vi "FS50_auto-tune_LV2019.vi"() -> ()   [LabVIEW 2019]
uses:
  C/Program Files (x86)/National Instruments/LabVIEW 2021/instr.lib/NKTP_API/NKTP_API.lvlib
panel:
  out "Auto-tune Status":string
  out "Current D4":dbl
  out "Current D3":dbl
  out "Current D2":dbl
  out "Connected":bool
  in  "Auto-tune":bool
  out "Auto-tune on":bool
  in  "Power Level":u16(slide) max=100 step=1 scale=0.0..100.0
  out "Emission On":bool
  in  "Emission":bool
  in  "VISA resource name":refnum<visa-resource-name>
  in  "Exit":bool
  in  "Connect":bool
  out "error out":errorcluster
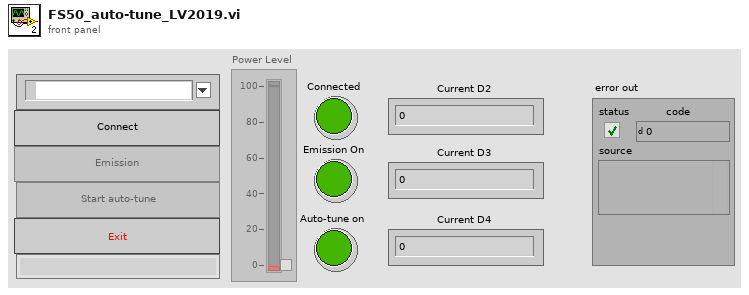
[diagram p1: front panel]
types:
  T1 = enum8{"Enabled", "Disabled", "Disabled and Grayed Out"}
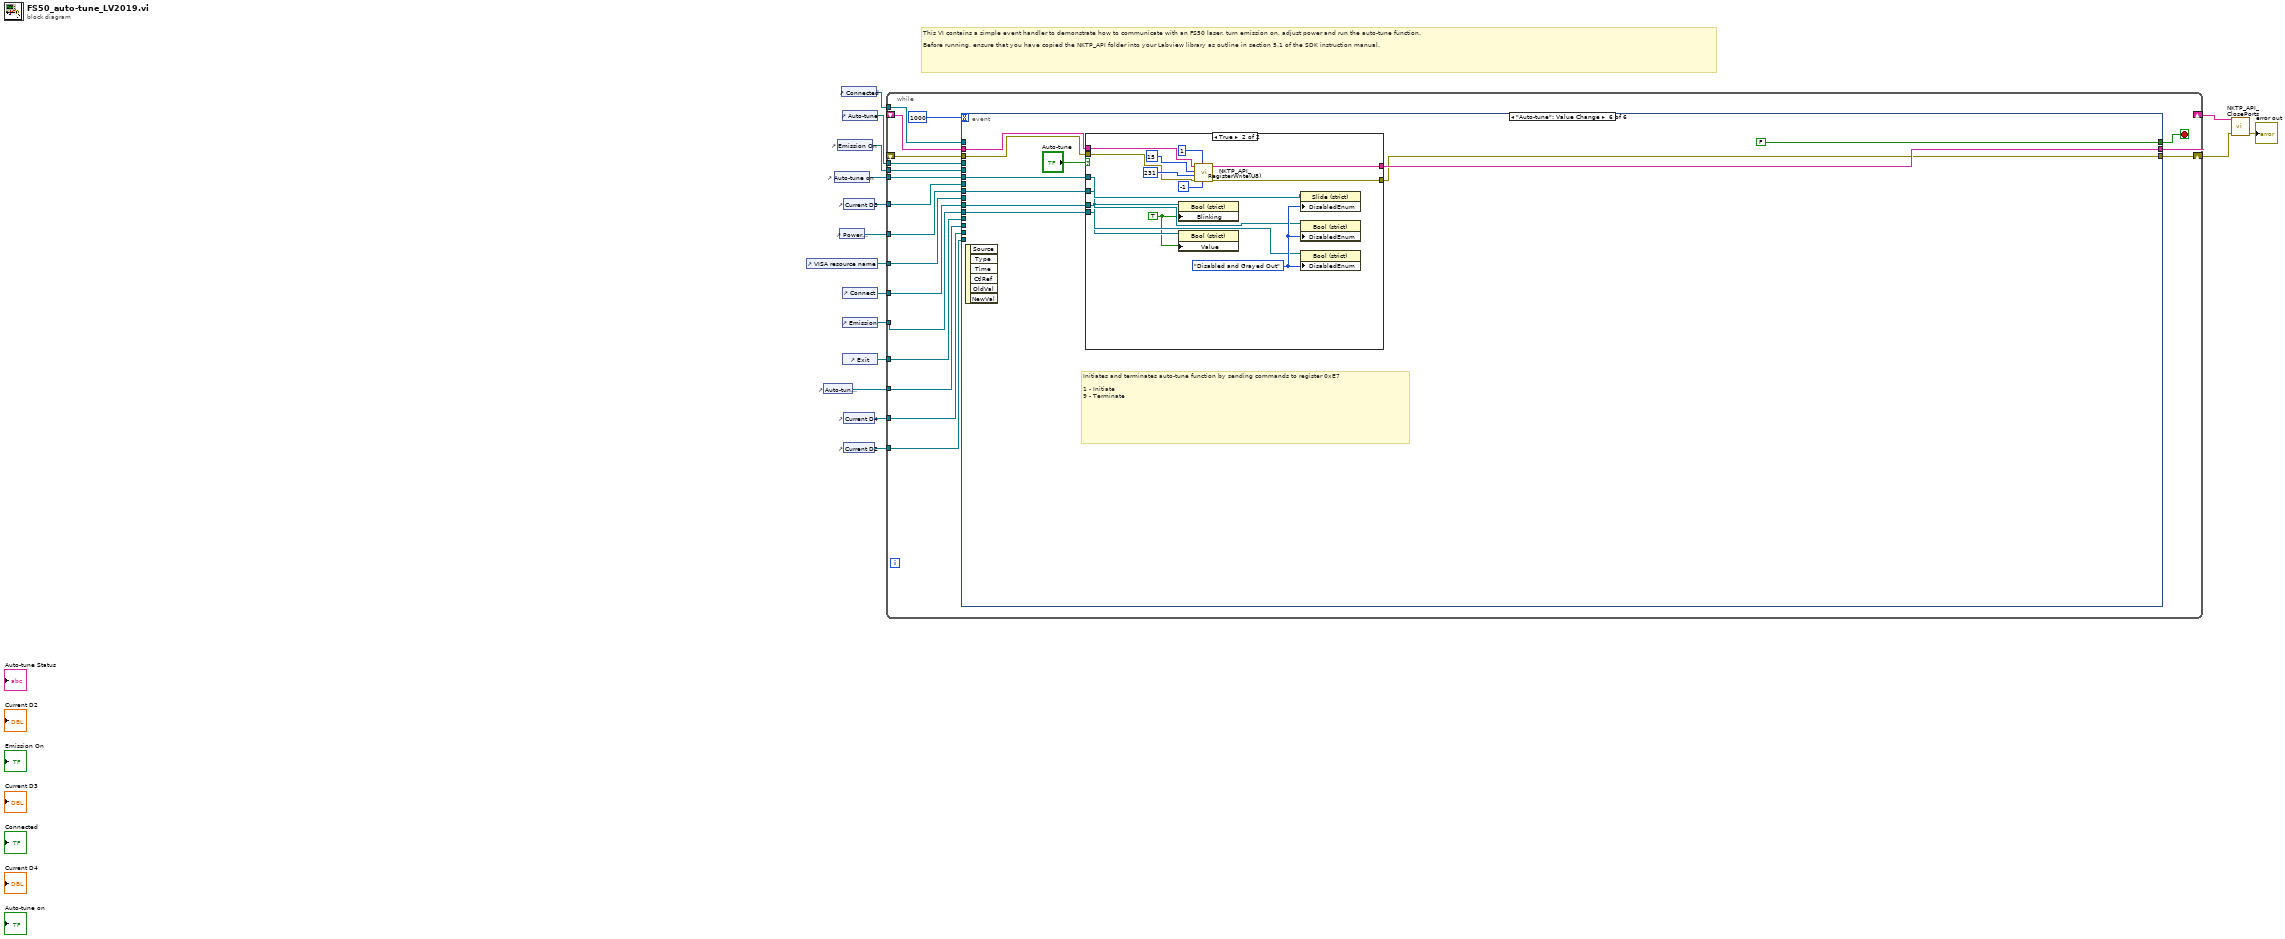
[diagram p0: block diagram]
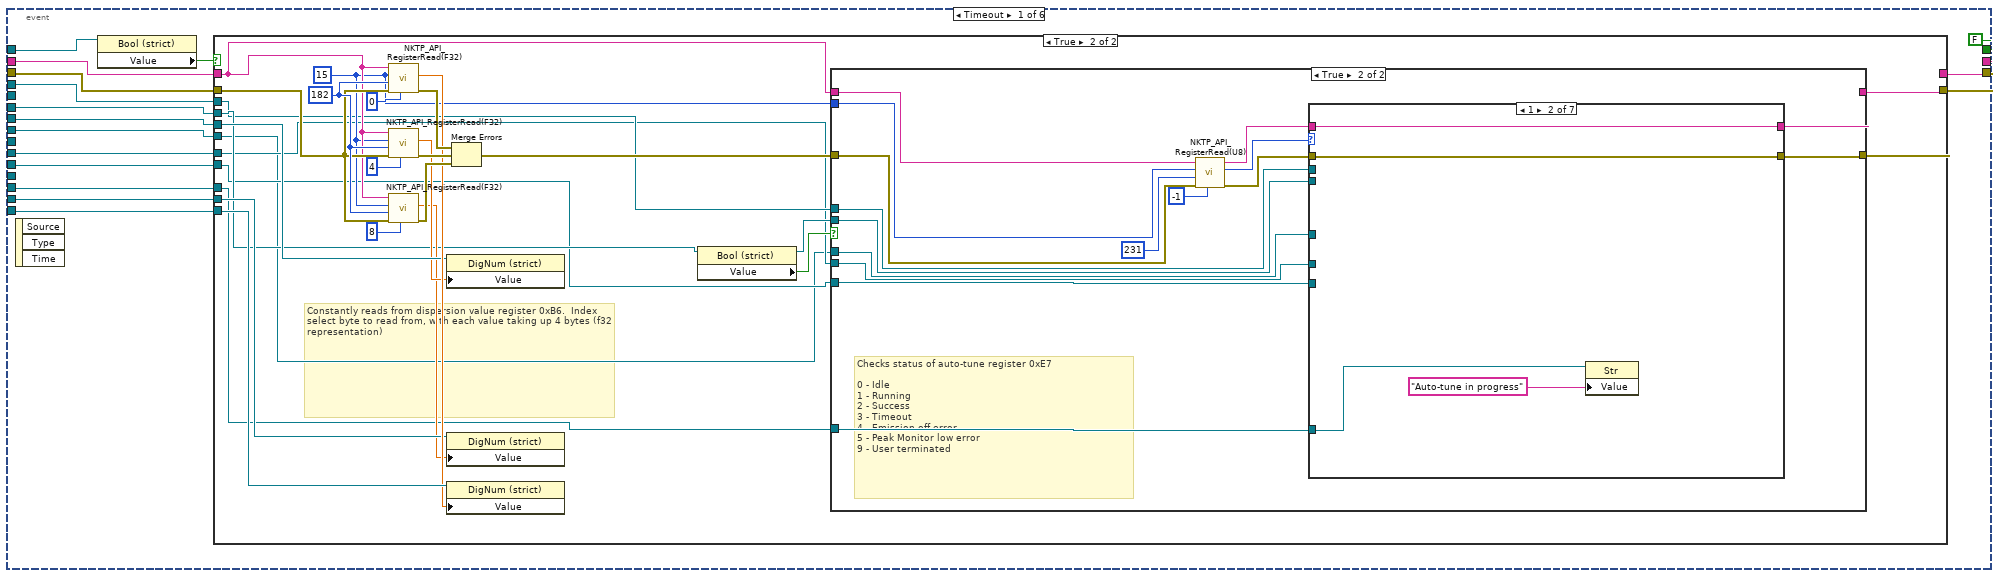
[diagram p2: hidden frame]
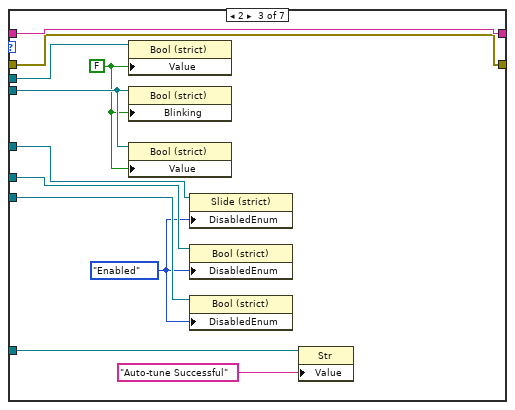
[diagram p6: hidden frame]
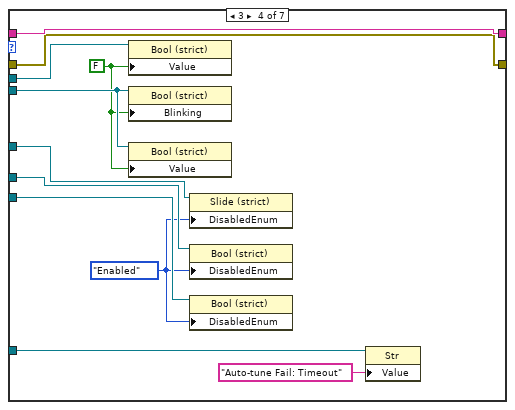
[diagram p7: hidden frame]
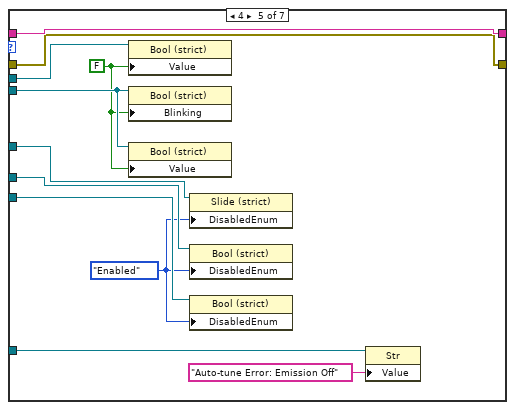
[diagram p8: hidden frame]
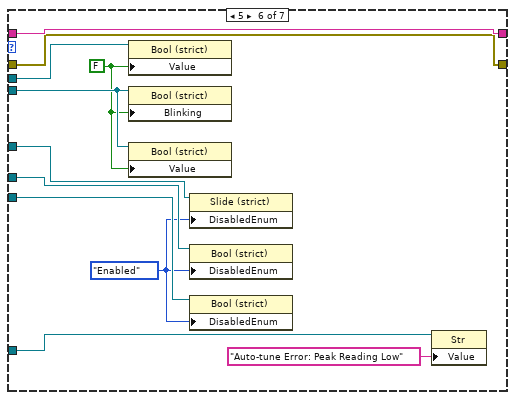
[diagram p9: hidden frame]
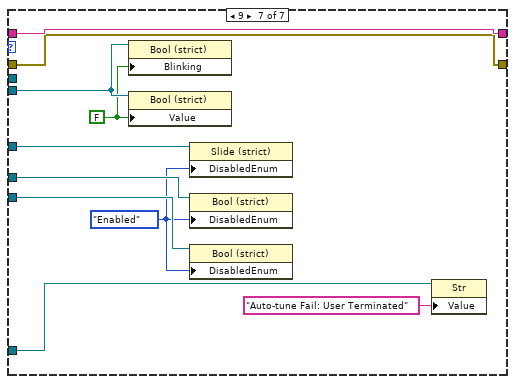
[diagram p10: hidden frame]
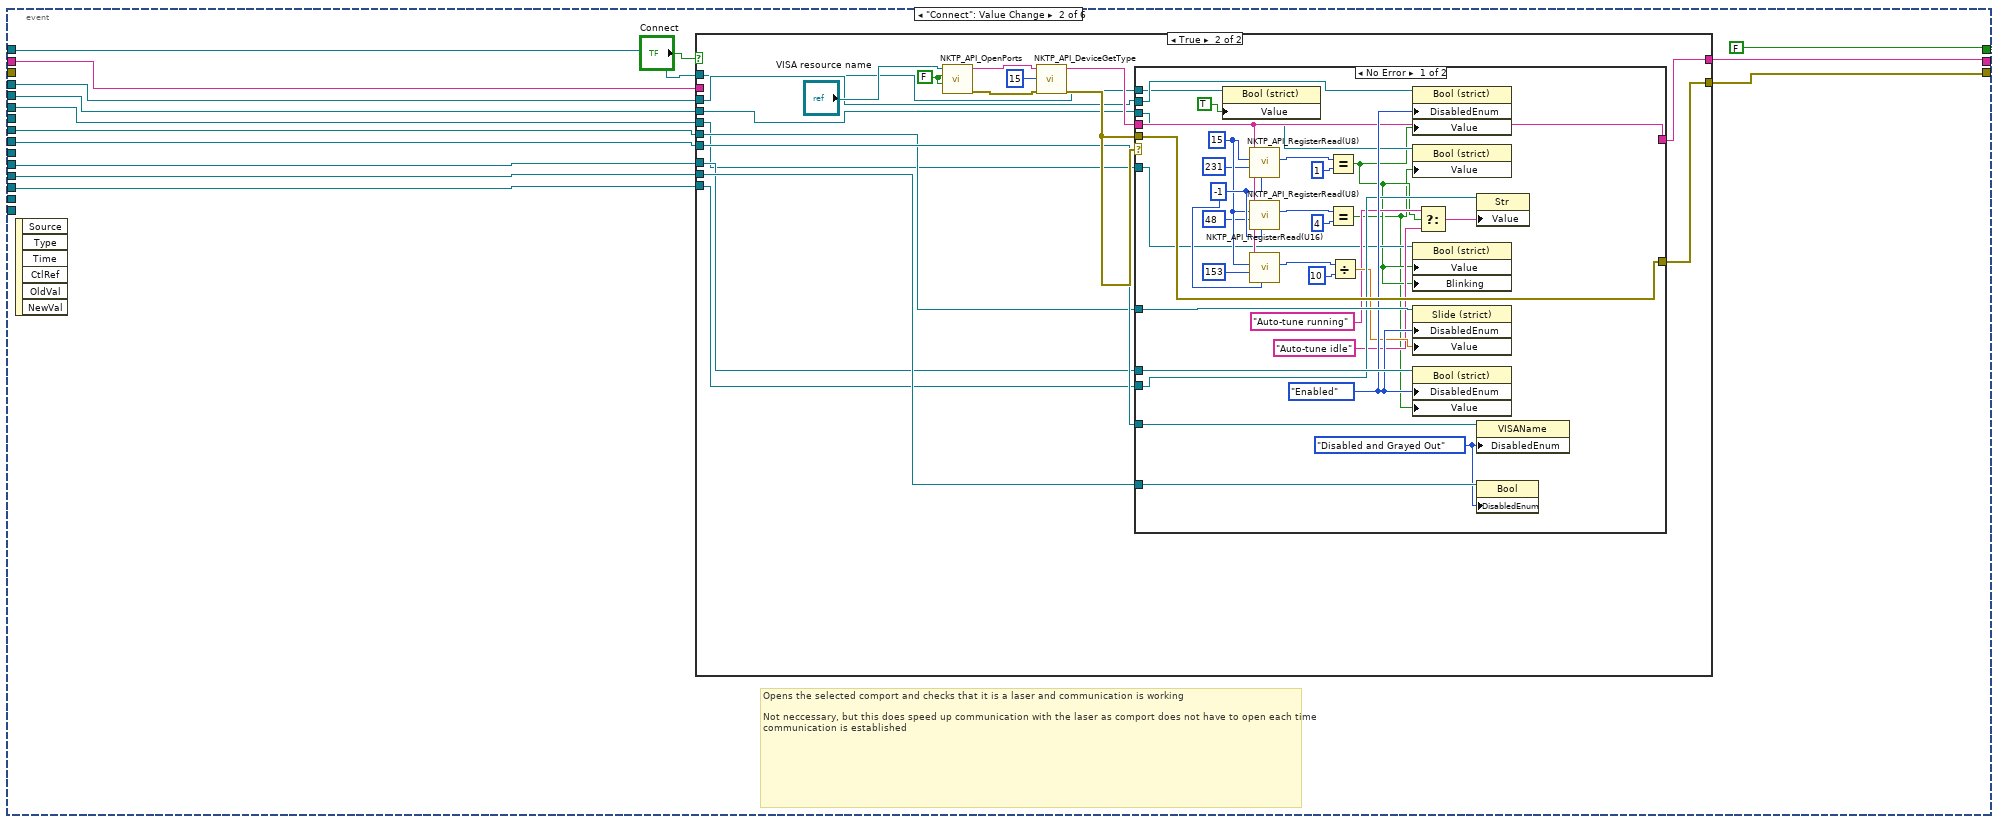
[diagram p11: hidden frame]
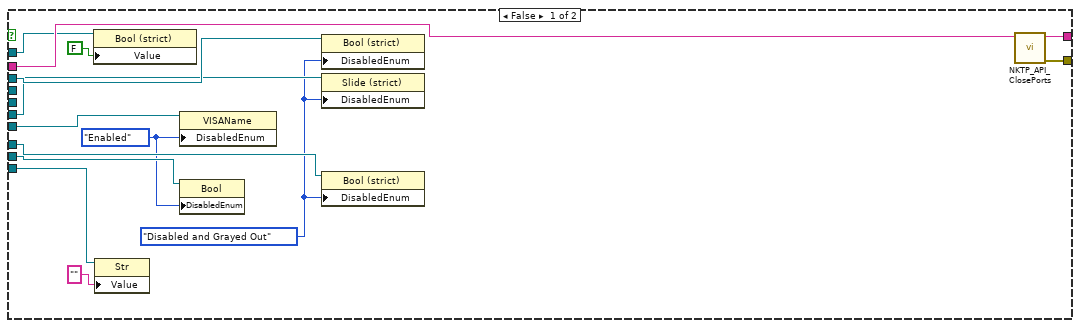
[diagram p12: hidden frame]
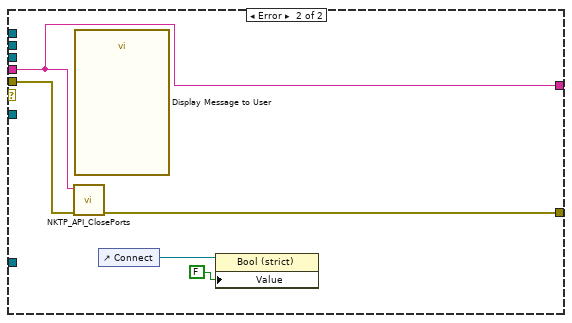
[diagram p13: hidden frame]
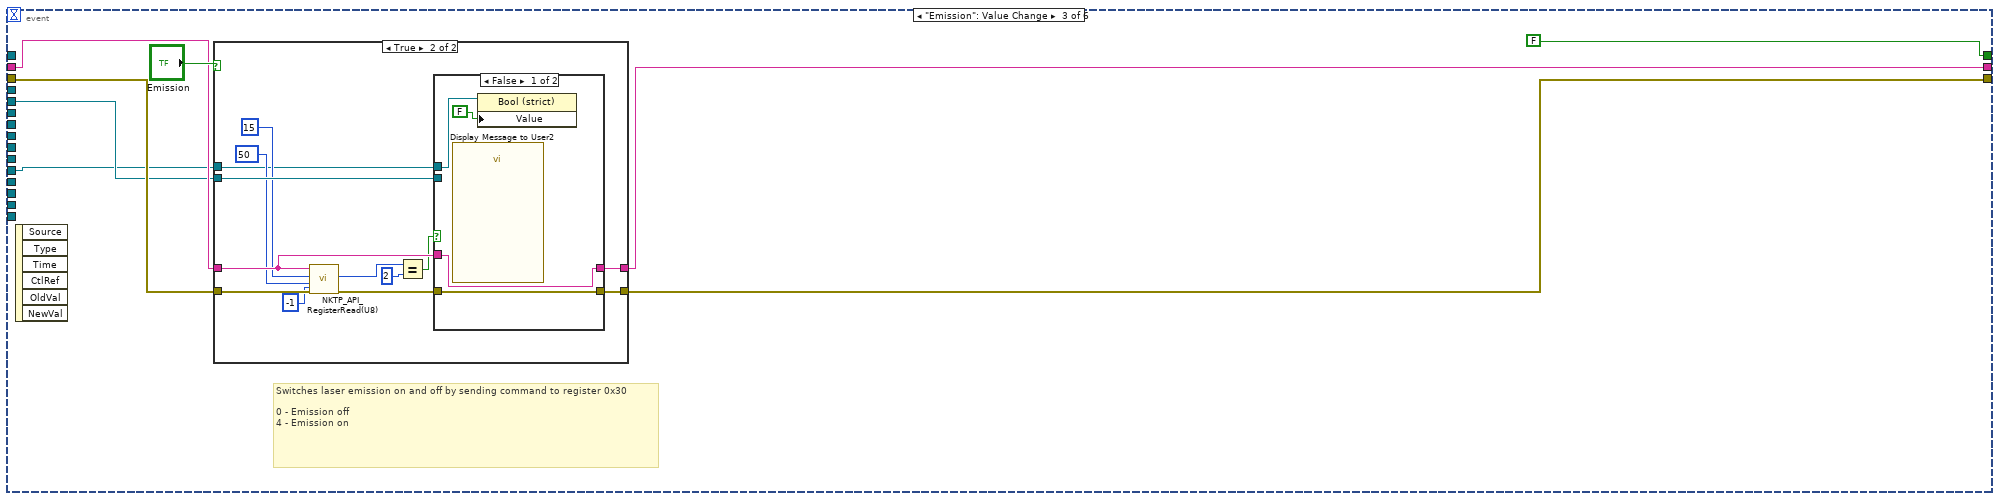
[diagram p14: hidden frame]
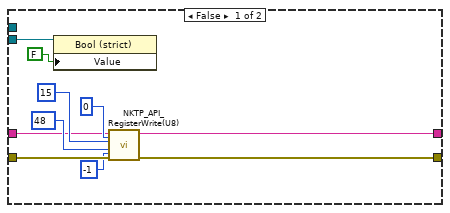
[diagram p15: hidden frame]
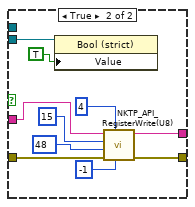
[diagram p16: hidden frame]
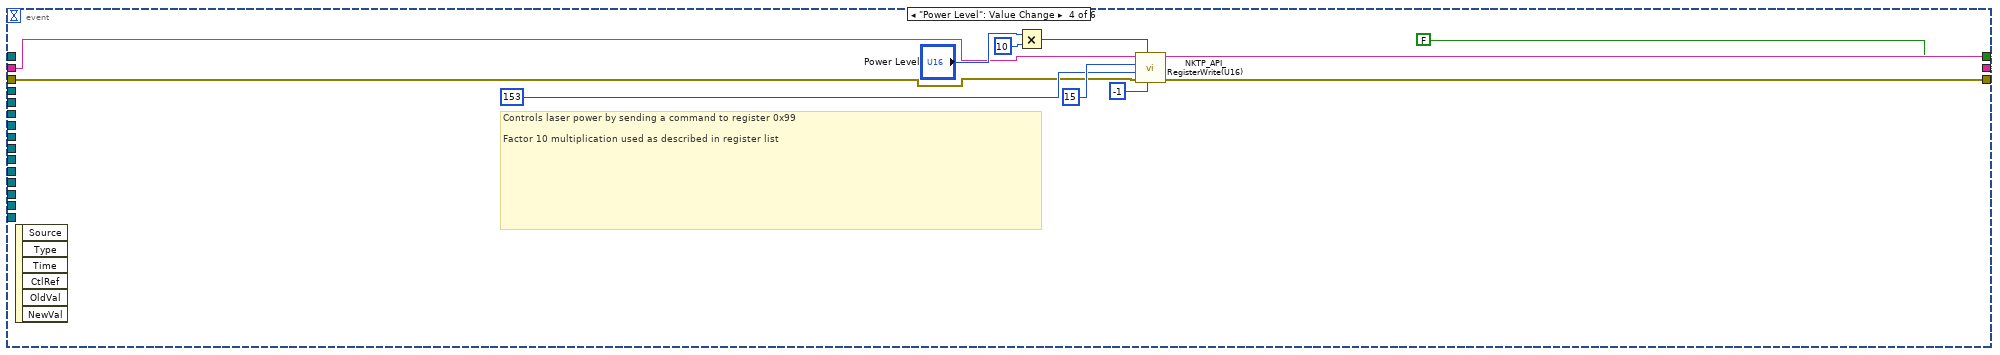
[diagram p17: hidden frame]
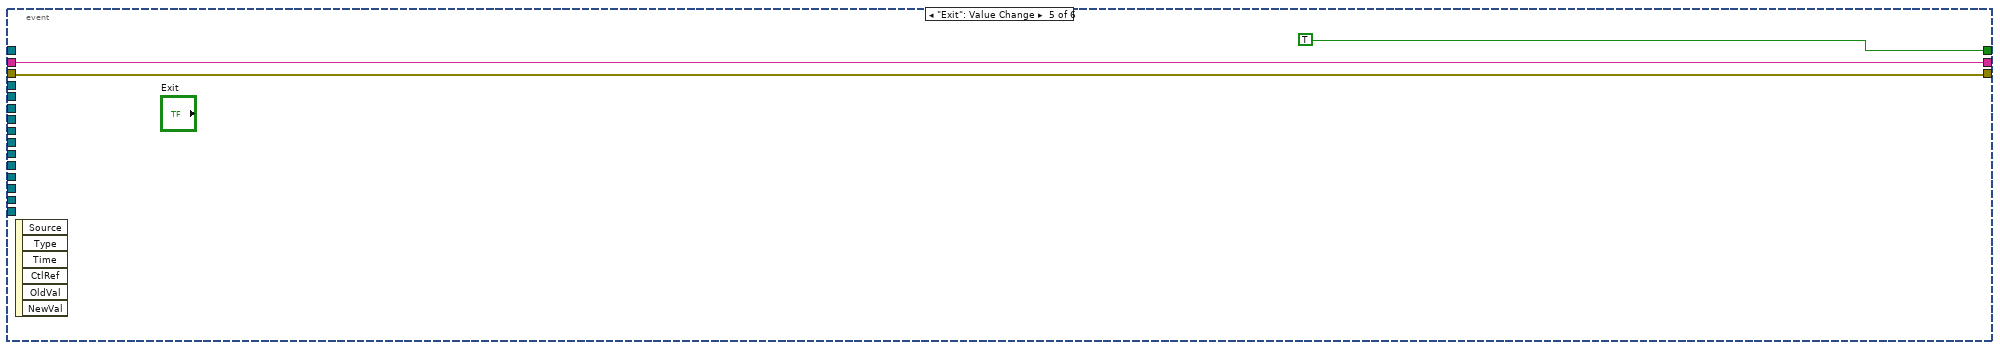
[diagram p18: hidden frame]
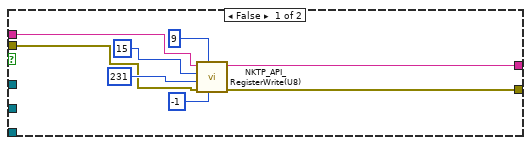
[diagram p19: hidden frame]
diagram:
  # "This VI contains a simple event handler to demonstrate how to communicate with an FS50 laser, turn emission on, adjust power and run the auto-tune function.\n\nBefore running, ensure that you have copied the NKTP_API folder into your Labview library as outline in section 5.1 of the SDK instruction manual."
  n1 = control-ref of="VISA resource name"() -> (w9:refnum<vi>)
  n2 = control-ref of="Auto-tune Status"() -> (w1:refnum<vi>)
  n3 = control-ref of="Auto-tune on"() -> (w13:refnum<vi>)
  n4 = control-ref of="Emission On"() -> (w7:refnum<vi>)
  n5 = control-ref of="Power Level"() -> (w10:refnum<vi>)
  n6 = control-ref of="Connected"() -> (w6:refnum<vi>)
  n7 = control-ref of="Auto-tune"() -> (w12:refnum<vi>)
  n8 = control-ref of="Connect"() -> (w2:refnum<vi>)
  n9 = control-ref of="Emission"() -> (w11:refnum<vi>)
  n10 = control-ref of="Exit"() -> (w8:refnum<vi>)
  n11 = control-ref of="Current D3"() -> (w4:refnum<vi>)
  n12 = control-ref of="Current D4"() -> (w3:refnum<vi>)
  n13 = control-ref of="Current D2"() -> (w5:refnum<vi>)
  n14 = while {
    shift-right: [w33] -> w14
    shift-left: _ -> [w30]
    shift-right: [w35] -> w16
    shift-left: _ -> [w32]
    tunnel: w13 -> [w29]
    tunnel: w12 -> [w28]
    tunnel: w11 -> [w27]
    tunnel: w10 -> [w26]
    tunnel: w9 -> [w25]
    tunnel: w8 -> [w24]
    tunnel: w7 -> [w23]
    tunnel: w6 -> [w22]
    tunnel: w5 -> [w21]
    tunnel: w4 -> [w20]
    tunnel: w3 -> [w19]
    tunnel: w2 -> [w18]
    tunnel: w1 -> [w17]
    stop <- w34 stop-if-true
    n15 = event shown="[5] \"Auto-tune\": Value Change" {
      selector: _ -> [_ _ _ _ _ _]
      dyn-events: _ -> [_ _ _ _ _ _]
      timeout: 1000 -> [_ _ _ _ _ _]
      tunnel: [w48 w172 w245 w289 w297 w301] -> w33
      tunnel: [w47 w171 w244 w290 w298 w303] -> w35
      tunnel: [FALSE FALSE FALSE FALSE TRUE FALSE] -> w34
      tunnel: w32 -> [w46 w168 w247 w293 w298 w307]
      tunnel: w30 -> [w51 _ w246 w288 w297 w302]
      tunnel: w29 -> [w42 w159 _ _ _ w308]
      tunnel: w28 -> [w40 w167 _ _ _ _]
      tunnel: w27 -> [w38 w166 w241 _ _ w306]
      tunnel: w26 -> [w37 w165 _ _ _ w304]
      tunnel: w25 -> [_ w164 _ _ _ _]
      tunnel: w24 -> [_ w163 _ _ _ _]
      tunnel: w23 -> [_ w160 w243 _ _ _]
      tunnel: w22 -> [w50 w162 _ _ _ _]
      tunnel: w21 -> [w45 _ _ _ _ _]
      tunnel: w20 -> [w44 _ _ _ _ _]
      tunnel: w19 -> [w43 _ _ _ _ _]
      tunnel: w18 -> [w39 _ _ _ _ w305]
      tunnel: w17 -> [w41 w161 _ _ _ _]
      event Timeout {
        n16 = event-data() -> ()  [unwired: 1 in, 3 out]
        n17 = property class="Bool (strict)"(reference=w50) -> ("Value"=w49:bool)  [unwired: 1 in, 2 out]
        n18 = case shown="True" w49 {
          tunnel: w51 -> [w53 w79]
          tunnel: [w53 w61] -> w48
          tunnel: [w52 w60] -> w47
          tunnel: w46 -> [w52 w64]
          tunnel: w45 -> [_ w72]
          tunnel: w44 -> [_ w70]
          tunnel: w43 -> [_ w68]
          tunnel: w42 -> [_ w66]
          tunnel: w41 -> [_ w59]
          tunnel: w40 -> [_ w57]
          tunnel: w39 -> [_ w56]
          tunnel: w38 -> [_ w55]
          tunnel: w37 -> [_ w54]
          frame False {
          }
          frame True {
            w80 = u8 182 ("regId")
            w63 = u8 15 ("devId")
            # "Constantly reads from dispersion value register 0xB6.  Index select byte to read from, with each value taking up 4 bytes (f32 representation)"
            n19 = call <instrlib>:"NKTP_API_RegisterRead(F32).vi"("index"=i16 0, "error in"=w79, "regId"=w80, "devId"=w63, "portname"=w64) -> ("error out"=w78:errorcluster, "value"=w71:sgl)  [unwired: 4 in, 1 out]
            n20 = call <instrlib>:"NKTP_API_RegisterRead(F32).vi"("index"=i16 4, "error in"=w79, "regId"=w80, "devId"=w63, "portname"=w64) -> ("error out"=w77:errorcluster, "value"=w69:sgl)  [unwired: 4 in, 1 out]
            n21 = call <instrlib>:"NKTP_API_RegisterRead(F32).vi"("index"=i16 8, "error in"=w79, "regId"=w80, "devId"=w63, "portname"=w64) -> ("error out"=w76:errorcluster, "value"=w67:sgl)  [unwired: 4 in, 1 out]
            n22 = property class="DigNum (strict)"(reference=w70, "Value"=w69) -> ()  [unwired: 1 in, 2 out]
            n23 = property class="DigNum (strict)"(reference=w68, "Value"=w67) -> ()  [unwired: 1 in, 2 out]
            n24 = property class="DigNum (strict)"(reference=w72, "Value"=w71) -> ()  [unwired: 1 in, 2 out]
            n25 = Merge Errors(w78, w77, w76) -> (w62:errorcluster)
            n26 = property class="Bool (strict)"(reference=w66) -> (reference out=w58:refnum<vi>, "Value"=w65:bool)  [unwired: 1 in, 1 out]
            n27 = case shown="True" w65 {
              tunnel: w64 -> [w81 w98]
              tunnel: w63 -> [_ w97]
              tunnel: w62 -> [w82 w94]
              tunnel: [w82 w88] -> w61
              tunnel: [w81 w90] -> w60
              tunnel: w59 -> [_ w92]
              tunnel: w58 -> [_ w87]
              tunnel: w57 -> [_ w86]
              tunnel: w56 -> [_ w85]
              tunnel: w55 -> [_ w84]
              tunnel: w54 -> [_ w83]
              frame False {
              }
              frame True {
                # "Checks status of auto-tune register 0xE7\n\n0 - Idle\n1 - Running\n2 - Success\n3 - Timeout\n4 - Emission off error\n5 - Peak Monitor low error\n9 - User terminated"
                n28 = call <instrlib>:"NKTP_API_RegisterRead(U8).vi"("index"=i16 -1, "error in"=w94, "regId"=u8 231, "devId"=w97, "portname"=w98) -> ("error out"=w89:errorcluster, "value"=w93:u8, "portname out"=w91:string)  [unwired: 4 in]
                n29 = case shown="1" w93 {
                  tunnel: w92 -> [_ w104 w115 w126 w137 w148 w158]
                  tunnel: w91 -> [w100 w102 w113 w124 w135 w146 w156]
                  tunnel: [w100 w102 w113 w124 w135 w146 w156] -> w90
                  tunnel: w89 -> [w99 w101 w112 w123 w134 w145 w155]
                  tunnel: [w99 w101 w112 w123 w134 w145 w155] -> w88
                  tunnel: w87 -> [_ _ w106 w117 w128 w139 w150]
                  tunnel: w86 -> [_ _ w111 w122 w133 w144 _]
                  tunnel: w85 -> [_ _ w110 w121 w132 w143 w154]
                  tunnel: w84 -> [_ _ w109 w120 w131 w142 w153]
                  tunnel: w83 -> [_ _ w108 w119 w130 w141 w152]
                  frame 0, Default {
                  }
                  frame 1 {
                    n30 = property class="Str"(reference=w104, "Value"="Auto-tune in progress") -> ()  [unwired: 1 in, 2 out]
                  }
                  frame 2 {
                    w107 = T1."Enabled" ("Disabled")
                    w105 = FALSE ("Value")
                    n31 = property class="Bool (strict)"(reference=w111, "Value"=w105) -> ()  [unwired: 1 in, 2 out]
                    n32 = property class="Bool (strict)"(reference=w106, "Blinking"=w105) -> ()  [unwired: 1 in, 2 out]
                    n33 = property class="Bool (strict)"(reference=w106, "Value"=w105) -> ()  [unwired: 1 in, 2 out]
                    n34 = property class="Slide (strict)"(reference=w108, "DisabledEnum"=w107) -> ()  [unwired: 1 in, 2 out]
                    n35 = property class="Bool (strict)"(reference=w110, "DisabledEnum"=w107) -> ()  [unwired: 1 in, 2 out]
                    n36 = property class="Bool (strict)"(reference=w109, "DisabledEnum"=w107) -> ()  [unwired: 1 in, 2 out]
                    n37 = property class="Str"(reference=w115, "Value"="Auto-tune Successful") -> ()  [unwired: 1 in, 2 out]
                  }
                  frame 3 {
                    w118 = T1."Enabled" ("Disabled")
                    w116 = FALSE ("Value")
                    n38 = property class="Bool (strict)"(reference=w122, "Value"=w116) -> ()  [unwired: 1 in, 2 out]
                    n39 = property class="Bool (strict)"(reference=w117, "Blinking"=w116) -> ()  [unwired: 1 in, 2 out]
                    n40 = property class="Bool (strict)"(reference=w117, "Value"=w116) -> ()  [unwired: 1 in, 2 out]
                    n41 = property class="Slide (strict)"(reference=w119, "DisabledEnum"=w118) -> ()  [unwired: 1 in, 2 out]
                    n42 = property class="Bool (strict)"(reference=w121, "DisabledEnum"=w118) -> ()  [unwired: 1 in, 2 out]
                    n43 = property class="Bool (strict)"(reference=w120, "DisabledEnum"=w118) -> ()  [unwired: 1 in, 2 out]
                    n44 = property class="Str"(reference=w126, "Value"="Auto-tune Fail: Timeout") -> ()  [unwired: 1 in, 2 out]
                  }
                  frame 4 {
                    w129 = T1."Enabled" ("Disabled")
                    w127 = FALSE ("Value")
                    n45 = property class="Bool (strict)"(reference=w133, "Value"=w127) -> ()  [unwired: 1 in, 2 out]
                    n46 = property class="Bool (strict)"(reference=w128, "Blinking"=w127) -> ()  [unwired: 1 in, 2 out]
                    n47 = property class="Bool (strict)"(reference=w128, "Value"=w127) -> ()  [unwired: 1 in, 2 out]
                    n48 = property class="Slide (strict)"(reference=w130, "DisabledEnum"=w129) -> ()  [unwired: 1 in, 2 out]
                    n49 = property class="Bool (strict)"(reference=w132, "DisabledEnum"=w129) -> ()  [unwired: 1 in, 2 out]
                    n50 = property class="Bool (strict)"(reference=w131, "DisabledEnum"=w129) -> ()  [unwired: 1 in, 2 out]
                    n51 = property class="Str"(reference=w137, "Value"="Auto-tune Error: Emission Off") -> ()  [unwired: 1 in, 2 out]
                  }
                  frame 5 {
                    w140 = T1."Enabled" ("Disabled")
                    w138 = FALSE ("Value")
                    n52 = property class="Bool (strict)"(reference=w144, "Value"=w138) -> ()  [unwired: 1 in, 2 out]
                    n53 = property class="Bool (strict)"(reference=w139, "Blinking"=w138) -> ()  [unwired: 1 in, 2 out]
                    n54 = property class="Bool (strict)"(reference=w139, "Value"=w138) -> ()  [unwired: 1 in, 2 out]
                    n55 = property class="Slide (strict)"(reference=w141, "DisabledEnum"=w140) -> ()  [unwired: 1 in, 2 out]
                    n56 = property class="Bool (strict)"(reference=w143, "DisabledEnum"=w140) -> ()  [unwired: 1 in, 2 out]
                    n57 = property class="Bool (strict)"(reference=w142, "DisabledEnum"=w140) -> ()  [unwired: 1 in, 2 out]
                    n58 = property class="Str"(reference=w148, "Value"="Auto-tune Error: Peak Reading Low") -> ()  [unwired: 1 in, 2 out]
                  }
                  frame 9 {
                    w151 = T1."Enabled" ("Disabled")
                    w149 = FALSE ("Value")
                    n59 = property class="Bool (strict)"(reference=w150, "Blinking"=w149) -> ()  [unwired: 1 in, 2 out]
                    n60 = property class="Bool (strict)"(reference=w150, "Value"=w149) -> ()  [unwired: 1 in, 2 out]
                    n61 = property class="Slide (strict)"(reference=w152, "DisabledEnum"=w151) -> ()  [unwired: 1 in, 2 out]
                    n62 = property class="Bool (strict)"(reference=w154, "DisabledEnum"=w151) -> ()  [unwired: 1 in, 2 out]
                    n63 = property class="Bool (strict)"(reference=w153, "DisabledEnum"=w151) -> ()  [unwired: 1 in, 2 out]
                    n64 = property class="Str"(reference=w158, "Value"="Auto-tune Fail: User Terminated") -> ()  [unwired: 1 in, 2 out]
                  }
                }
              }
            }
          }
        }
      }
      event "Connect": Value Change {
        # "Opens the selected comport and checks that it is a laser and communication is working\n\nNot neccessary, but this does speed up communication with the laser as comport does not have to open each time communication is established"
        n65 = event-data() -> ()  [unwired: 1 in, 6 out]
        n66 = case shown="True" "Connect" {
          tunnel: [w186 w204] -> w172
          tunnel: [w185 w203] -> w171
          tunnel: w168 -> [w184 _]
          tunnel: w164 -> [w183 w195]
          tunnel: w163 -> [w182 w194]
          tunnel: w166 -> [w181 w193]
          tunnel: w167 -> [w180 w192]
          tunnel: w165 -> [w179 w191]
          tunnel: w162 -> [w176 w190]
          tunnel: w161 -> [w174 w189]
          tunnel: w160 -> [_ w188]
          tunnel: w159 -> [_ w187]
          frame False {
            w177 = T1."Disabled and Grayed Out" ("Disabled")
            w178 = T1."Enabled" ("Disabled")
            n67 = property class="Bool (strict)"(reference=w176, "Value"=FALSE) -> ()  [unwired: 1 in, 2 out]
            n68 = property class="Str"(reference=w174, "Value"="") -> ()  [unwired: 1 in, 2 out]
            n69 = property class="VISAName"(reference=w183, "DisabledEnum"=w178) -> ()  [unwired: 1 in, 2 out]
            n70 = property class="Bool"(reference=w182, "DisabledEnum"=w178) -> ()  [unwired: 1 in, 2 out]
            n71 = property class="Bool (strict)"(reference=w180, "DisabledEnum"=w177) -> ()  [unwired: 1 in, 2 out]
            n72 = property class="Slide (strict)"(reference=w179, "DisabledEnum"=w177) -> ()  [unwired: 1 in, 2 out]
            n73 = property class="Bool (strict)"(reference=w181, "DisabledEnum"=w177) -> ()  [unwired: 1 in, 2 out]
            n74 = call <instrlib>:"NKTP_API_ClosePorts.vi"("portnames"=w184) -> ("error out"=w186:errorcluster, "portnames out"=w185:string)  [unwired: 9 in]
          }
          frame True {
            w202 = FALSE ("AutoMode")
            n75 = call <instrlib>:"NKTP_API_OpenPorts.vi"("liveMode"=w202, "autoMode"=w202, "portnames"="VISA resource name") -> ("error out"=w199:errorcluster, "portnames out"=w198:string)  [unwired: 7 in]
            n76 = call <instrlib>:"NKTP_API_DeviceGetType.vi"("error in"=w199, "devId"=u8 15, "portname"=w198) -> ("error out"=w200:errorcluster, "portname"=w201:string)  [unwired: 6 in, 1 out]
            n77 = case shown="No Error" w200 {
              tunnel: w200 -> [w235 w237]
              tunnel: [w235 w236] -> w204
              tunnel: w201 -> [w224 w238]
              tunnel: [w224 w238] -> w203
              tunnel: w195 -> [w234 _]
              tunnel: w194 -> [w233 _]
              tunnel: w193 -> [w232 _]
              tunnel: w192 -> [w231 _]
              tunnel: w191 -> [w230 _]
              tunnel: w190 -> [w227 _]
              tunnel: w189 -> [w225 _]
              tunnel: w188 -> [w208 _]
              tunnel: w187 -> [w207 _]
              frame No Error {
                w222 = u8 15 ("devId")
                w223 = i16 -1 ("index")
                w229 = T1."Enabled" ("Disabled")
                w228 = T1."Disabled and Grayed Out" ("Disabled")
                n78 = property class="Bool (strict)"(reference=w227, "Value"=TRUE) -> ()  [unwired: 1 in, 2 out]
                n79 = call <instrlib>:"NKTP_API_RegisterRead(U8).vi"("index"=w223, "regId"=u8 231, "devId"=w222, "portname"=w224) -> ("value"=w216:u8)  [unwired: 5 in, 2 out]
                n80 = call <instrlib>:"NKTP_API_RegisterRead(U8).vi"("index"=w223, "regId"=u8 48, "devId"=w222, "portname"=w224) -> ("value"=w218:u8)  [unwired: 5 in, 2 out]
                n81 = call <instrlib>:"NKTP_API_RegisterRead(U16).vi"("index"=w223, "regId"=u8 153, "devId"=w222, "portname"=w224) -> ("value"=w214:u16)  [unwired: 5 in, 2 out]
                n82 = Equal?(x=w216, y=u8 1) -> (x = y?=w206:bool)
                n83 = Equal?(x=w218, y=u8 4) -> (x = y?=w205:bool)
                n84 = Divide(x=w214, y=u16 10) -> (x/y=w212:dbl)
                n85 = property class="Bool (strict)"(reference=w231, "DisabledEnum"=w229, "Value"=w206) -> ()  [unwired: 1 in, 2 out]
                n86 = property class="Bool (strict)"(reference=w208, "Value"=w205) -> ()  [unwired: 1 in, 2 out]
                n87 = property class="Bool (strict)"(reference=w207, "Value"=w206, "Blinking"=w206) -> ()  [unwired: 1 in, 2 out]
                n88 = property class="Slide (strict)"(reference=w230, "DisabledEnum"=w229, "Value"=w212) -> ()  [unwired: 1 in, 2 out]
                n89 = property class="Bool (strict)"(reference=w232, "DisabledEnum"=w229, "Value"=w205) -> ()  [unwired: 1 in, 2 out]
                n90 = Select(t="Auto-tune running", s=w206, f="Auto-tune idle" ("Value")) -> (s? t:f=w210:string)
                n91 = property class="Str"(reference=w225, "Value"=w210) -> ()  [unwired: 1 in, 2 out]
                n92 = property class="VISAName"(reference=w234, "DisabledEnum"=w228) -> ()  [unwired: 1 in, 2 out]
                n93 = property class="Bool"(reference=w233, "DisabledEnum"=w228) -> ()  [unwired: 1 in, 2 out]
              }
              frame Error {
                n94 = call <instrlib>:"NKTP_API_ClosePorts.vi"("error in"=w237, "portnames"=w238) -> ("error out"=w236:errorcluster)  [unwired: 8 in, 1 out]
                n95 = call "Display Message to User"() -> ()  [unwired: 10 in, 2 out]
                n96 = control-ref of="Connect"() -> (w240:refnum<vi>)
                n97 = property class="Bool (strict)"(reference=w240, "Value"=FALSE) -> ()  [unwired: 1 in, 2 out]
              }
            }
          }
        }
      }
      event "Emission": Value Change {
        # "Switches laser emission on and off by sending command to register 0x30\n\n0 - Emission off\n4 - Emission on"
        n98 = event-data() -> ()  [unwired: 1 in, 6 out]
        n99 = case shown="True" "Emission" {
          tunnel: w243 -> [w258 w271]
          tunnel: w247 -> [w253 w268]
          tunnel: w246 -> [w252 w267]
          tunnel: [w251 w270] -> w245
          tunnel: [w250 w269] -> w244
          tunnel: w241 -> [_ w259]
          frame False {
            n100 = property class="Bool (strict)"(reference=w258, "Value"=FALSE) -> ()  [unwired: 1 in, 2 out]
            n101 = call <instrlib>:"NKTP_API_RegisterWrite(U8).vi"("index"=i16 -1, "value"=u8 0, "error in"=w252, "regId"=u8 48, "devId"=u8 15, "portname"=w253) -> ("error out"=w251:errorcluster, "portname out"=w250:string)  [unwired: 4 in]
          }
          frame True {
            n102 = call <instrlib>:"NKTP_API_RegisterRead(U8).vi"("index"=i16 -1, "error in"=w267, "regId"=u8 50, "devId"=u8 15, "portname"=w268) -> ("error out"=w266:errorcluster, "value"=w262:u8)  [unwired: 4 in, 1 out]
            n103 = Equal?(x=w262, y=u8 2) -> (x = y?=w260:bool)
            n104 = case shown="False" w260 {
              tunnel: w271 -> [_ w285]
              tunnel: w268 -> [w275 w283]
              tunnel: w266 -> [w274 w279]
              tunnel: [w274 w278] -> w270
              tunnel: [w275 w277] -> w269
              tunnel: w259 -> [w273 _]
              frame False {
                n105 = call "Display Message to User2"() -> ()  [unwired: 10 in, 2 out]
                n106 = property class="Bool (strict)"(reference=w273, "Value"=FALSE) -> ()  [unwired: 1 in, 2 out]
              }
              frame True {
                n107 = property class="Bool (strict)"(reference=w285, "Value"=TRUE ("Emission On")) -> ()  [unwired: 1 in, 2 out]
                n108 = call <instrlib>:"NKTP_API_RegisterWrite(U8).vi"("index"=i16 -1, "value"=u8 4, "error in"=w279, "regId"=u8 48, "devId"=u8 15, "portname"=w283) -> ("error out"=w278:errorcluster, "portname out"=w277:string)  [unwired: 4 in]
              }
            }
          }
        }
      }
      event "Power Level": Value Change {
        # "Controls laser power by sending a command to register 0x99\n\nFactor 10 multiplication used as described in register list"
        n109 = event-data() -> ()  [unwired: 1 in, 6 out]
        n110 = Multiply(x="Power Level", y=u16 10) -> (x*y=w294:u16)
        n111 = call <instrlib>:"NKTP_API_RegisterWrite(U16).vi"("index"=i16 -1, "value"=w294, "error in"=w288, "regId"=u8 153, "devId"=u8 15, "portname"=w293) -> ("error out"=w289:errorcluster, "portname out"=w290:string)  [unwired: 4 in]
      }
      event "Exit": Value Change {
        n112 = event-data() -> ()  [unwired: 1 in, 6 out]
      }
      event "Auto-tune": Value Change {
        # "Initiates and terminates auto-tune function by sending commands to register 0xE7\n\n1 - Initiate\n9 - Terminate"
        n113 = event-data() -> ()  [unwired: 1 in, 6 out]
        n114 = case shown="True" "Auto-tune" {
          tunnel: w308 -> [_ w322]
          tunnel: w307 -> [w317 w331]
          tunnel: w306 -> [_ w323]
          tunnel: w305 -> [_ w325]
          tunnel: w304 -> [_ w324]
          tunnel: [w312 w320] -> w303
          tunnel: w302 -> [w311 w319]
          tunnel: [w310 w318] -> w301
          frame False {
            n115 = call <instrlib>:"NKTP_API_RegisterWrite(U8).vi"("index"=i16 -1, "value"=u8 9, "error in"=w311, "regId"=u8 231, "devId"=u8 15, "portname"=w317) -> ("error out"=w310:errorcluster, "portname out"=w312:string)  [unwired: 4 in]
          }
          frame True {
            w326 = T1."Disabled and Grayed Out" ("Disabled")
            w321 = TRUE ("Value")
            n116 = property class="Bool (strict)"(reference=w322, "Blinking"=w321) -> ()  [unwired: 1 in, 2 out]
            n117 = property class="Bool (strict)"(reference=w322, "Value"=w321) -> ()  [unwired: 1 in, 2 out]
            n118 = call <instrlib>:"NKTP_API_RegisterWrite(U8).vi"("index"=i16 -1, "value"=u8 1, "error in"=w319, "regId"=u8 231, "devId"=u8 15, "portname"=w331) -> ("error out"=w318:errorcluster, "portname out"=w320:string)  [unwired: 4 in]
            n119 = property class="Slide (strict)"(reference=w324, "DisabledEnum"=w326) -> ()  [unwired: 1 in, 2 out]
            n120 = property class="Bool (strict)"(reference=w325, "DisabledEnum"=w326) -> ()  [unwired: 1 in, 2 out]
            n121 = property class="Bool (strict)"(reference=w323, "DisabledEnum"=w326) -> ()  [unwired: 1 in, 2 out]
          }
        }
      }
    }
  }
  n122 = call <instrlib>:"NKTP_API_ClosePorts.vi"("error in"=w14, "portnames"=w16) -> ("error out"=→"error out":errorcluster)  [unwired: 8 in, 1 out]
